vi "Heater_D2XX_updated.vi"(8 "error in (no error)":errorcluster, 11 "Numeric 2":i32) -> (0 "error out":errorcluster)   [LabVIEW 2019]
uses:
  <userlib>/LevyLab/D2XX-LV/private/Open Device (index).vi
  <instrlib>/FTDI/D2XX/FT_Open_Device_By_Index.vi
  <userlib>/LevyLab/D2XX-LV/private/FT_Status to Error.vi
  <userlib>/LevyLab/D2XX-LV/private/Write Data (String).vi
  <userlib>/LevyLab/D2XX-LV/D2XX-lv.lvlib
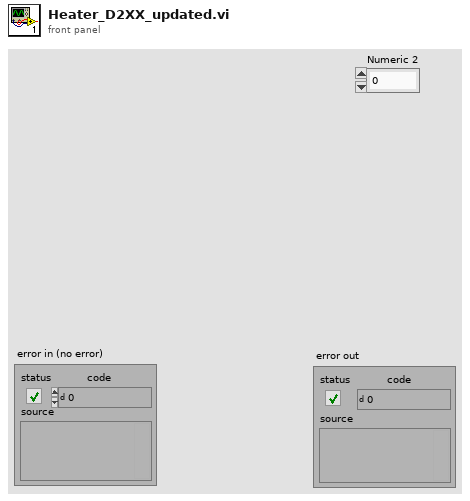
[diagram p1: front panel]
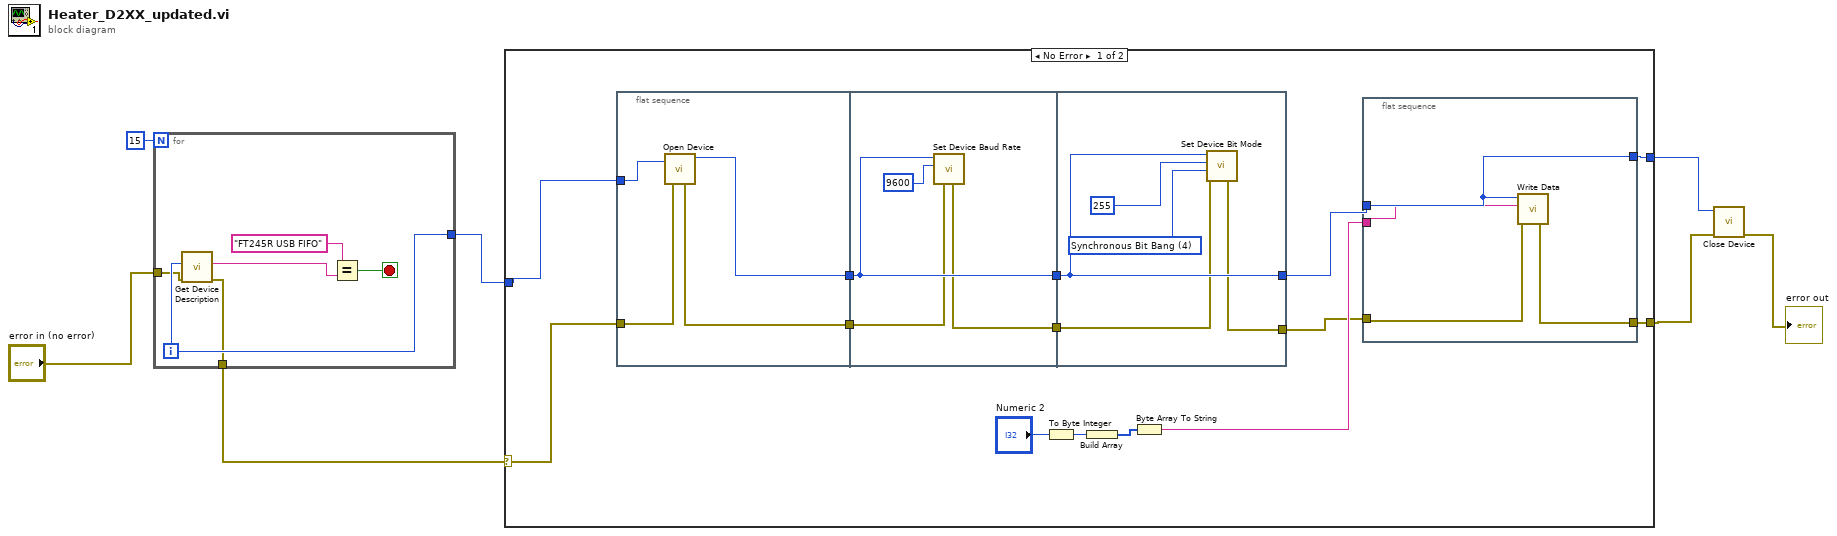
[diagram p0: block diagram]
diagram:
  n1 = for {
    N: 15 -> [_]
    tunnel: [w10] -> w6
    tunnel: "error in (no error)" -> [w9]
    tunnel: [w8] -> w4
    i -> [w10]
    stop <- w12 stop-if-true
    n2 = call <userlib>:"Get Device Description.vi"("error in (no error)"=w9, "Device Index"=w10) -> ("error out"=w8:errorcluster, "Device Description"=w11:string)  [unwired: 8 in]
    n3 = Equal?(x="FT245R USB FIFO", y=w11) -> (x = y?=w12:bool)
  }
  n4 = case shown="No Error" w4 {
    selector: w4 -> [w18 w45]
    tunnel: [w21 w46] -> w3
    tunnel: [w14 w45] -> w2
    tunnel: w6 -> [w22 w46]
    frame No Error {
      n5 = flat-sequence {
        tunnel: w22 -> [w31]
        tunnel: [w30] -> w20
        tunnel: w18 -> [w29]
        tunnel: [w28] -> w17
        tunnel: w20 -> [w34]
        tunnel: [w34] -> w19
        tunnel: w17 -> [w33]
        tunnel: [w32] -> w16
        tunnel: [w40] -> w24
        tunnel: w19 -> [w40]
        tunnel: w16 -> [w39]
        tunnel: [w36] -> w15
        frame #0 {
          n6 = call-poly <userlib>:"Open Device.vi"("error in (no error)"=w29, "Device Index"=w31) -> ("error out"=w28:errorcluster, "Handle"=w30:u32)  [unwired: 8 in]
        }
        frame #1 {
          n7 = call <userlib>:"Set Device Baud Rate.vi"("error in (no error)"=w33, "Baud Rate"=u32 9600, "Handle"=w34) -> ("error out"=w32:errorcluster)  [unwired: 7 in, 1 out]
        }
        frame #2 {
          w37 = u8 4 items=["Reset Bit Mode"=0, "Asynchronous Bit Bang"=1, "MPSSE"=2, "Synchronous Bit Bang"=4, "MCU Host Bus Emulation"=8, "Fast Opto-Isolated Serial"=16, "CBUS Bit Bang"=32, "Single Channel 245 Synchronous FIFO"=64] ("Bit Mode")
          n8 = call <userlib>:"Set Device Bit Mode.vi"("error in (no error)"=w39, "Bit Mode"=w37, "Bit Mode Mask"=u8 255, "Handle"=w40) -> ("error out"=w36:errorcluster)  [unwired: 6 in, 1 out]
        }
      }
      n9 = To Byte Integer(number="Numeric 2") -> (8bit integer=w27:i8)
      n10 = Build Array(w27) -> (w26:i8[])
      n11 = Byte Array To String(unsigned byte array=w26) -> (string=w25:string)
      n12 = flat-sequence {
        tunnel: w24 -> [w42]
        tunnel: [w42] -> w21
        tunnel: w25 -> [w41]
        tunnel: w15 -> [w44]
        tunnel: [w43] -> w14
        frame #0 {
          n13 = call-poly <userlib>:"Write Data.vi"("error in (no error)"=w44, "Write Buffer"=w41, "Handle"=w42) -> ("error out"=w43:errorcluster)  [unwired: 6 in, 2 out]
        }
      }
    }
    frame Error {
    }
  }
  n14 = call <userlib>:"Close Device.vi"("error in (no error)"=w2, "Handle"=w3) -> ("error out"=→"error out":errorcluster)  [unwired: 9 in]
